vi "Byte_to_DeviceConfigType.vi"(4 "Byte Array":u8[](array[numeric])) -> (1 "output cluster":T1)   [LabVIEW 2016]
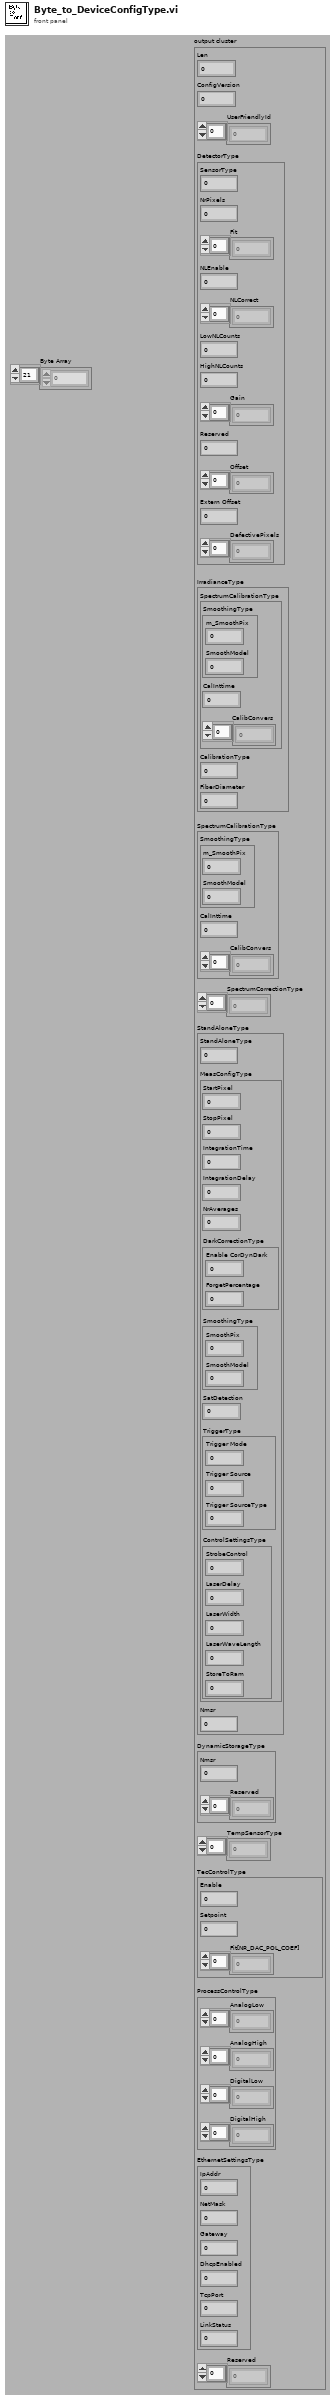
[diagram p1: front panel]
types:
  T1 = cluster{"Len":u16, "ConfigVersion":u16, "UserFriendlyId":u8[], "DetectorType":cluster{"SensorType":u8, "NrPixels":u16, "Fit":sgl[], "NLEnable":u8, "NLCorrect":dbl[], "LowNLCounts":dbl, "HighNLCounts":dbl, "Gain":sgl[], "Reserved":sgl, "Offset":sgl[], "Extern Offset":sgl, "DefectivePixels":u16[]}, "IrradianceType":cluster{"SpectrumCalibrationType":cluster{"SmoothingType":cluster{"m_SmoothPix":u16, "SmoothModel":u8}, "CalInttime":sgl, "CalibConvers":sgl[]}, "CalibrationType":u8, "FiberDiameter":i32}, "SpectrumCalibrationType":cluster{"SmoothingType":cluster{"m_SmoothPix":u16, "SmoothModel":u8}, "CalInttime":sgl, "CalibConvers":sgl[]}, "SpectrumCorrectionType":sgl[], "StandAloneType":cluster{"StandAloneType":u8, "MeasConfigType":cluster{"StartPixel":u16, "StopPixel":u16, "IntegrationTime":sgl, "IntegrationDelay":u32, "NrAverages":u32, "DarkCorrectionType":cluster{"Enable CorDynDark":u8, "ForgetPercentage":u8}, "SmoothingType":cluster{"SmoothPix":u16, "SmoothModel":u8}, "SatDetection":u8, "TriggerType":cluster{"Trigger Mode":u8, "Trigger Source":u8, "Trigger SourceType":u8}, "ControlSettingsType":cluster{"StrobeControl":u16, "LaserDelay":u32, "LaserWidth":u32, "LaserWaveLength":sgl, "StoreToRam":u16}}, "Nmsr":i16}, "DynamicStorageType":cluster{"Nmsr":i32, "Reserved":u8[]}, "TempSensorType":sgl[], "TecControlType":cluster{"Enable":u8, "Setpoint":sgl, "Fit[NR_DAC_POL_COEF]":sgl[]}, "ProcessControlType":cluster{"AnalogLow":sgl[], "AnalogHigh":sgl[], "DigitalLow":sgl[], "DigitalHigh":sgl[]}, "EthernetSettingsType":cluster{"IpAddr":u32, "NetMask":u32, "Gateway":u32, "DhcpEnabled":u8, "TcpPort":u16, "LinkStatus":u8}, "Reserved":u8[]}
  T2 = cluster{"Len":u16, "ConfigVersion":u16, "UserFriendlyId":u8[], "DetectorType":cluster{"SensorType":u8, "NrPixels":u16, "Fit":sgl[], "NLEnable":u8, "NLCorrect":dbl[], "LowNLCounts":dbl, "HighNLCounts":dbl, "Gain":sgl[], "Reserved":sgl, "Offset":sgl[], "Extern Offset":sgl, "DefectivePixels":u16[]}, "IrradianceType":cluster{"SpectrumCalibrationType":cluster{"SmoothingType":cluster{"m_SmoothPix":u16, "SmoothModel":u8}, "CalInttime":sgl, "CalibConvers":sgl[]}, "CalibrationType":u8, "FiberDiameter":i32}, "SpectrumCalibrationType":cluster{"SmoothingType":cluster{"m_SmoothPix":u16, "SmoothModel":u8}, "CalInttime":sgl, "CalibConvers":sgl[]}, "SpectrumCorrectionType":sgl[], "StandAloneType":cluster{"StandAloneType":u8, "MeasConfigType":cluster{"StartPixel":u16, "StopPixel":u16, "IntegrationTime":sgl, "IntegrationDelay":u32, "NrAverages":u32, "DarkCorrectionType":cluster{"Enable CorDynDark":u8, "ForgetPercentage":u8}, "SmoothingType":cluster{"SmoothPix":u16, "SmoothModel":u8}, "SatDetection":u8, "TriggerType":cluster{"Trigger Mode":u8, "Trigger Source":u8, "Trigger SourceType":u8}, "ControlSettingsType":cluster{"StrobeControl":u16, "LaserDelay":u32, "LaserWidth":u32, "LaserWaveLength":sgl, "StoreToRam":u16}}, "Nmsr":i16}, "DynamicStorageType":cluster{"Nmsr":i32, "Reserved":u8[]}, "TempSensorType":sgl[], "TecControlType":cluster{"Enable":u8, "Setpoint":sgl, "Fit[NR_DAC_POL_COEF]":sgl[]}, "ProcessControlType\n":cluster{"AnalogLow":sgl[], "AnalogHigh":sgl[], "DigitalLow":sgl[], "DigitalHigh":sgl[]}, "EthernetSettingsType":cluster{"IpAddr":u32, "NetMask":u32, "Gateway":u32, "DhcpEnabled":u8, "TcpPort":u16, "LinkStatus":u8}, "Reserved":u8[]}
  T3 = cluster{u8, u16, sgl[], u8, dbl[], dbl, dbl, sgl[], sgl, sgl[], sgl, u16[]}
  T4 = cluster{cluster{cluster{u16, u8}, sgl, sgl[]}, u8, i32}
  T5 = cluster{u16, u16, sgl, u32, u32, cluster{u8, u8}, cluster{u16, u8}, u8, cluster{u8, u8, u8}, cluster{u16, u32, u32, sgl, u16}}
  T6 = cluster{u8, cluster{u16, u16, sgl, u32, u32, cluster{u8, u8}, cluster{u16, u8}, u8, cluster{u8, u8, u8}, cluster{u16, u32, u32, sgl, u16}}, i16}
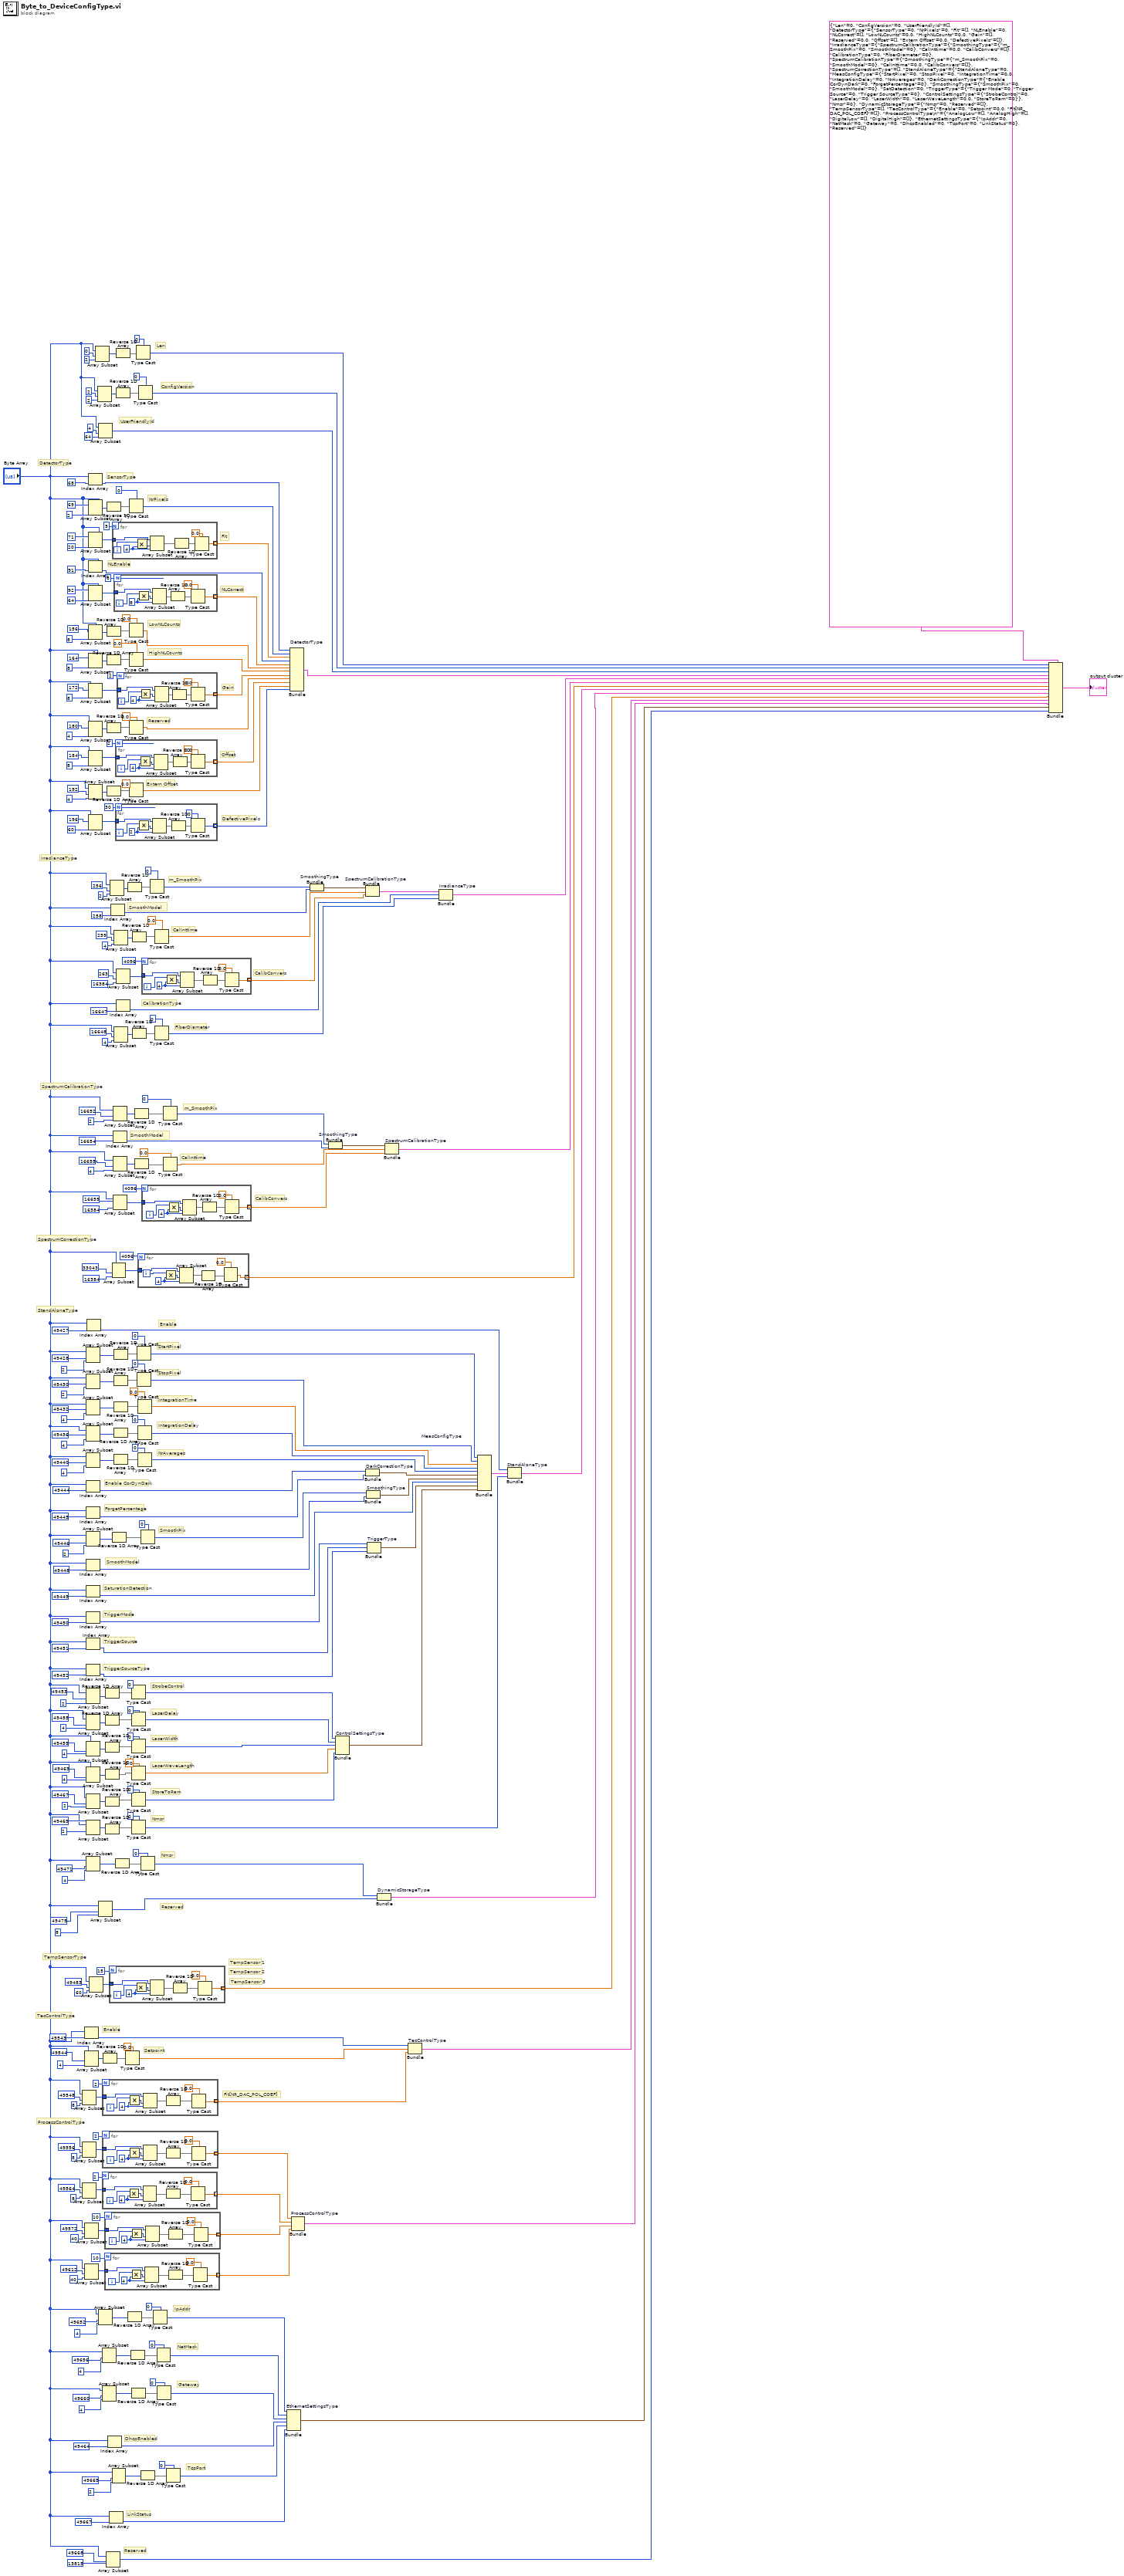
[diagram p0: block diagram]
diagram:
  # "Enable"
  # "LinkStatus"
  # "DhcpEnabled"
  # "TcpPort"
  # "Gateway"
  # "NetMask"
  # "IpAddr"
  # "ProcessControlType"
  # "TecControlType"
  # "Len"
  # "ConfigVersion"
  # "Fit[NR_DAC_POL_COEF]"
  # "Setpoint"
  # "Enable"
  # "UserFriendlyId"
  # "SensorType"
  # "NrPixels"
  # "Fit"
  # "NLEnable"
  # "NLCorrect"
  # "LowNLCounts"
  # "HighNLCounts"
  # "Gain"
  # "Offset"
  # "DetectorType"
  # "TempSensor 3"
  # "TempSensor 2"
  # "Reserved"
  # "TempSensor 1"
  # "TempSensorType"
  # "Reserved"
  # "Nmsr"
  # "Nmsr"
  # "StoreToRam"
  # "LaserWaveLength"
  # "LaserWidth"
  # "LaserDelay"
  # "StrobeControl"
  # "TriggerSourceType"
  # "TriggerSource"
  # "TriggerMode"
  # "SaturationDetection"
  # "SmoothModel"
  # "SmoothPix"
  # "ForgetPercentage"
  # "Enable CorDynDark"
  # "NrAverages"
  # "IntegrationDelay"
  # "IntegrationTime"
  # "StopPixel"
  # "StartPixel"
  # "StandAloneType"
  # "SpectrumCorrectionType"
  # "CalibConvers"
  # "CalInttime"
  # "SmoothModel"
  # "m_SmoothPix"
  # "SpectrumCalibrationType"
  # "FiberDiameter"
  # "CalibrationType"
  # "CalibConvers"
  # "CalInttime"
  # "SmoothModel"
  # "IrradianceType"
  # "m_SmoothPix"
  # "DefectivePixels"
  # "Reserved"
  # "Extern Offset"
  n1 = Array Subset(array="Byte Array", index=49564, length=8) -> (w59:u8[])
  n2 = Array Subset(array="Byte Array", index=49548, length=8) -> (w68:u8[])
  n3 = Array Subset(array="Byte Array", index=49556, length=8) -> (w63:u8[])
  n4 = Index Array(array="Byte Array", index=49543 ("length")) -> (element=w75:u8)
  n5 = Array Subset(array="Byte Array", index=49612, length=40) -> (w51:u8[])
  n6 = Array Subset(array="Byte Array", index=49544, length=4) -> (w71:u8[])
  n7 = Array Subset(array="Byte Array", index=49572, length=40) -> (w55:u8[])
  n8 = Array Subset(array="Byte Array", index=49471 ("length"), length=4) -> (w42:u8[])
  n9 = Array Subset(array="Byte Array", index=49428, length=2) -> (w219:u8[])
  n10 = Array Subset(array="Byte Array", index=49430, length=2) -> (w214:u8[])
  n11 = Array Subset(array="Byte Array", index=49432, length=4) -> (w211:u8[])
  n12 = Array Subset(array="Byte Array", index=49436, length=4) -> (w202:u8[])
  n13 = Array Subset(array="Byte Array", index=49440, length=4) -> (w199:u8[])
  n14 = Index Array(array="Byte Array", index=49444 ("length")) -> (element=w94:u8)
  n15 = Index Array(array="Byte Array", index=49445 ("length")) -> (element=w93:u8)
  n16 = Array Subset(array="Byte Array", index=49446, length=2) -> (w193:u8[])
  n17 = Index Array(array="Byte Array", index=49448 ("length")) -> (element=w91:u8)
  n18 = Index Array(array="Byte Array", index=49449 ("length")) -> (element=w90:u8)
  n19 = Index Array(array="Byte Array", index=49450 ("length")) -> (element=w89:u8)
  n20 = Index Array(array="Byte Array", index=49451 ("length")) -> (element=w88:u8)
  n21 = Index Array(array="Byte Array", index=49452 ("length")) -> (element=w87:u8)
  n22 = Array Subset(array="Byte Array", index=49453, length=2) -> (w181:u8[])
  n23 = Array Subset(array="Byte Array", index=49455, length=4) -> (w178:u8[])
  n24 = Array Subset(array="Byte Array", index=49459, length=4) -> (w171:u8[])
  n25 = Array Subset(array="Byte Array", index=49463, length=4) -> (w168:u8[])
  n26 = Array Subset(array="Byte Array", index=49467, length=2) -> (w161:u8[])
  n27 = Array Subset(array="Byte Array", index=49469, length=2) -> (w156:u8[])
  n28 = Index Array(array="Byte Array", index=49427 ("length")) -> (element=w100:u8)
  n29 = Index Array(array="Byte Array", index=68 ("length")) -> (element=w133:u8)
  n30 = Array Subset(array="Byte Array", index=69, length=2) -> (w297:u8[])
  n31 = Array Subset(array="Byte Array", index=71, length=20) -> (w130:u8[])
  n32 = Index Array(array="Byte Array", index=91 ("length")) -> (element=w129:u8)
  n33 = Array Subset(array="Byte Array", index=92, length=64) -> (w127:u8[])
  n34 = Array Subset(array="Byte Array", index=156, length=8) -> (w283:u8[])
  n35 = Array Subset(array="Byte Array", index=164, length=8) -> (w280:u8[])
  n36 = Array Subset(array="Byte Array", index=172, length=8) -> (w123:u8[])
  n37 = Array Subset(array="Byte Array", index=180, length=4) -> (w271:u8[])
  n38 = Array Subset(array="Byte Array", index=184, length=8) -> (w120:u8[])
  n39 = Array Subset(array="Byte Array", index=192, length=4) -> (w263:u8[])
  n40 = Array Subset(array="Byte Array", index=196, length=60) -> (w118:u8[])
  n41 = Array Subset(array="Byte Array", index=49483, length=60) -> (w78:u8[])
  n42 = Array Subset(array="Byte Array", index=0, length=2) -> (w302:u8[])
  n43 = Array Subset(array="Byte Array", index=2, length=2) -> (w301:u8[])
  n44 = Array Subset(array="Byte Array", index=4, length=64) -> (w134:u8[])
  n45 = Array Subset(array="Byte Array", index=49475, length=8) -> (w77:u8[])
  n46 = Array Subset(array="Byte Array", index=49652 ("length"), length=4) -> (w35:u8[])
  n47 = for {
    N: 2 -> [_]
    tunnel: w59 -> [w315]
    tunnel: [w313] -> w46 mode=indexing
    i -> [w316]
    w317 = 4 ("length")
    n48 = Multiply(x=w316, y=w317) -> (x*y=w318:i32)
    n49 = Array Subset(array=w315, index=w318, length=w317) -> (w311:u8[])
    n50 = Reverse 1D Array(array=w311) -> (reversed array=w312:u8[])
    n51 = Type Cast(type=sgl 0.0, x=w312) -> (*(type *) &x=w313:sgl)
  }
  n52 = Array Subset(array="Byte Array", index=49656 ("length"), length=4) -> (w30:u8[])
  n53 = for {
    N: 2 -> [_]
    tunnel: w68 -> [w323]
    tunnel: [w321] -> w64 mode=indexing
    i -> [w324]
    w325 = 4 ("length")
    n54 = Multiply(x=w324, y=w325) -> (x*y=w326:i32)
    n55 = Array Subset(array=w323, index=w326, length=w325) -> (w319:u8[])
    n56 = Reverse 1D Array(array=w319) -> (reversed array=w320:u8[])
    n57 = Type Cast(type=sgl 0.0, x=w320) -> (*(type *) &x=w321:sgl)
  }
  n58 = for {
    N: 2 -> [_]
    tunnel: w63 -> [w331]
    tunnel: [w329] -> w47 mode=indexing
    i -> [w332]
    w333 = 4 ("length")
    n59 = Multiply(x=w332, y=w333) -> (x*y=w334:i32)
    n60 = Array Subset(array=w331, index=w334, length=w333) -> (w327:u8[])
    n61 = Reverse 1D Array(array=w327) -> (reversed array=w328:u8[])
    n62 = Type Cast(type=sgl 0.0, x=w328) -> (*(type *) &x=w329:sgl)
  }
  n63 = Array Subset(array="Byte Array", index=49660 ("length"), length=4) -> (w25:u8[])
  n64 = Reverse 1D Array(array=w71) -> (reversed array=w70:u8[])
  n65 = for {
    N: 10 -> [_]
    tunnel: w51 -> [w339]
    tunnel: [w337] -> w44 mode=indexing
    i -> [w340]
    w341 = 4 ("length")
    n66 = Multiply(x=w340, y=w341) -> (x*y=w342:i32)
    n67 = Array Subset(array=w339, index=w342, length=w341) -> (w335:u8[])
    n68 = Reverse 1D Array(array=w335) -> (reversed array=w336:u8[])
    n69 = Type Cast(type=sgl 0.0, x=w336) -> (*(type *) &x=w337:sgl)
  }
  n70 = for {
    N: 10 -> [_]
    tunnel: w55 -> [w347]
    tunnel: [w345] -> w45 mode=indexing
    i -> [w348]
    w349 = 4 ("length")
    n71 = Multiply(x=w348, y=w349) -> (x*y=w350:i32)
    n72 = Array Subset(array=w347, index=w350, length=w349) -> (w343:u8[])
    n73 = Reverse 1D Array(array=w343) -> (reversed array=w344:u8[])
    n74 = Type Cast(type=sgl 0.0, x=w344) -> (*(type *) &x=w345:sgl)
  }
  n75 = Reverse 1D Array(array=w181) -> (reversed array=w180:u8[])
  n76 = Reverse 1D Array(array=w178) -> (reversed array=w179:u8[])
  n77 = Reverse 1D Array(array=w171) -> (reversed array=w170:u8[])
  n78 = Reverse 1D Array(array=w168) -> (reversed array=w169:u8[])
  n79 = Reverse 1D Array(array=w161) -> (reversed array=w162:u8[])
  n80 = Reverse 1D Array(array=w156) -> (reversed array=w155:u8[])
  n81 = Array Subset(array="Byte Array", index=49668, length=13815) -> (w7:u8[])
  n82 = Reverse 1D Array(array=w297) -> (reversed array=w298:u8[])
  n83 = Reverse 1D Array(array=w283) -> (reversed array=w282:u8[])
  n84 = Reverse 1D Array(array=w280) -> (reversed array=w281:u8[])
  n85 = Reverse 1D Array(array=w271) -> (reversed array=w270:u8[])
  n86 = Reverse 1D Array(array=w263) -> (reversed array=w264:u8[])
  n87 = Index Array(array="Byte Array", index=49464 ("length")) -> (element=w10:u8)
  n88 = for {
    N: 15 -> [_]
    tunnel: w78 -> [w355]
    tunnel: [w353] -> w3 mode=indexing
    i -> [w356]
    w357 = 4 ("length")
    n89 = Multiply(x=w356, y=w357) -> (x*y=w358:i32)
    n90 = Array Subset(array=w355, index=w358, length=w357) -> (w351:u8[])
    n91 = Reverse 1D Array(array=w351) -> (reversed array=w352:u8[])
    n92 = Type Cast(type=sgl 0.0, x=w352) -> (*(type *) &x=w353:sgl)
  }
  n93 = Index Array(array="Byte Array", index=49667 ("length")) -> (element=w8:u8)
  n94 = Array Subset(array="Byte Array", index=256, length=2) -> (w254:u8[])
  n95 = Index Array(array="Byte Array", index=258 ("length")) -> (element=w115:u8)
  n96 = for {
    N: 5 -> [_]
    tunnel: w130 -> [w363]
    tunnel: [w361] -> w131 mode=indexing
    i -> [w364]
    w365 = 4 ("length")
    n97 = Multiply(x=w364, y=w365) -> (x*y=w366:i32)
    n98 = Array Subset(array=w363, index=w366, length=w365) -> (w360:u8[])
    n99 = Reverse 1D Array(array=w360) -> (reversed array=w359:u8[])
    n100 = Type Cast(type=sgl 0.0, x=w359) -> (*(type *) &x=w361:sgl)
  }
  n101 = Array Subset(array="Byte Array", index=33043, length=16384) -> (w86:u8[])
  n102 = Array Subset "Array Subset"(array="Byte Array", index=49665 ("length"), length=2) -> (w17:u8[])
  n103 = Reverse 1D Array(array=w193) -> (reversed array=w194:u8[])
  n104 = Array Subset(array="Byte Array", index=16652, length=2) -> (w228:u8[])
  n105 = Index Array(array="Byte Array", index=16654 ("length")) -> (element=w107:u8)
  n106 = Array Subset(array="Byte Array", index=16655, length=4) -> (w231:u8[])
  n107 = Array Subset(array="Byte Array", index=16659, length=16384) -> (w85:u8[])
  n108 = Reverse 1D Array(array=w219) -> (reversed array=w220:u8[])
  n109 = Reverse 1D Array(array=w214) -> (reversed array=w213:u8[])
  n110 = Reverse 1D Array(array=w211) -> (reversed array=w212:u8[])
  n111 = Reverse 1D Array(array=w202) -> (reversed array=w201:u8[])
  n112 = Reverse 1D Array(array=w199) -> (reversed array=w200:u8[])
  n113 = for {
    N: 8 -> [_]
    tunnel: w127 -> [w371]
    tunnel: [w369] -> w128 mode=indexing
    i -> [w372]
    w373 = 8 ("length")
    n114 = Multiply(x=w372, y=w373) -> (x*y=w374:i32)
    n115 = Array Subset(array=w371, index=w374, length=w373) -> (w368:u8[])
    n116 = Reverse 1D Array(array=w368) -> (reversed array=w367:u8[])
    n117 = Type Cast(type=0.0, x=w367) -> (*(type *) &x=w369:dbl)
  }
  n118 = Array Subset(array="Byte Array", index=259, length=4) -> (w250:u8[])
  n119 = Array Subset(array="Byte Array", index=16648, length=4) -> (w241:u8[])
  n120 = for {
    N: 30 -> [_]
    tunnel: w118 -> [w379]
    tunnel: [w377] -> w117 mode=indexing
    i -> [w380]
    w381 = 2 ("length")
    n121 = Multiply(x=w380, y=w381) -> (x*y=w382:i32)
    n122 = Array Subset(array=w379, index=w382, length=w381) -> (w376:u8[])
    n123 = Reverse 1D Array(array=w376) -> (reversed array=w375:u8[])
    n124 = Type Cast(type=u16 0, x=w375) -> (*(type *) &x=w377:u16)
  }
  n125 = Reverse 1D Array(array=w42) -> (reversed array=w43:u8[])
  n126 = for {
    N: 2 -> [_]
    tunnel: w120 -> [w387]
    tunnel: [w385] -> w121 mode=indexing
    i -> [w388]
    w389 = 4 ("length")
    n127 = Multiply(x=w388, y=w389) -> (x*y=w390:i32)
    n128 = Array Subset(array=w387, index=w390, length=w389) -> (w384:u8[])
    n129 = Reverse 1D Array(array=w384) -> (reversed array=w383:u8[])
    n130 = Type Cast(type=sgl 0.0, x=w383) -> (*(type *) &x=w385:sgl)
  }
  n131 = Array Subset(array="Byte Array", index=263, length=16384) -> (w113:u8[])
  n132 = Reverse 1D Array(array=w302) -> (reversed array=w145:u8[])
  n133 = Reverse 1D Array(array=w301) -> (reversed array=w300:u8[])
  n134 = Index Array(array="Byte Array", index=16647 ("length")) -> (element=w111:u8)
  n135 = for {
    N: 2 -> [_]
    tunnel: w123 -> [w395]
    tunnel: [w393] -> w124 mode=indexing
    i -> [w396]
    w397 = 4 ("length")
    n136 = Multiply(x=w396, y=w397) -> (x*y=w398:i32)
    n137 = Array Subset(array=w395, index=w398, length=w397) -> (w392:u8[])
    n138 = Reverse 1D Array(array=w392) -> (reversed array=w391:u8[])
    n139 = Type Cast(type=sgl 0.0, x=w391) -> (*(type *) &x=w393:sgl)
  }
  n140 = Type Cast(type=sgl 0.0, x=w70) -> (*(type *) &x=w69:sgl)
  n141 = Reverse 1D Array(array=w35) -> (reversed array=w36:u8[])
  n142 = Reverse 1D Array(array=w254) -> (reversed array=w253:u8[])
  n143 = Type Cast(type=u16 0, x=w298) -> (*(type *) &x=w132:u16)
  n144 = Type Cast(type=0.0, x=w282) -> (*(type *) &x=w126:dbl)
  n145 = Type Cast(type=0.0, x=w281) -> (*(type *) &x=w125:dbl)
  n146 = Type Cast(type=sgl 0.0, x=w270) -> (*(type *) &x=w122:sgl)
  n147 = Type Cast(type=sgl 0.0, x=w264) -> (*(type *) &x=w119:sgl)
  n148 = Reverse 1D Array(array=w30) -> (reversed array=w31:u8[])
  n149 = Type Cast(type=u16 0, x=w180) -> (*(type *) &x=w84:u16)
  n150 = Type Cast(type=u32 0, x=w179) -> (*(type *) &x=w83:u32)
  n151 = Type Cast(type=u32 0, x=w170) -> (*(type *) &x=w82:u32)
  n152 = Type Cast(type=sgl 0.0, x=w169) -> (*(type *) &x=w81:sgl)
  n153 = Type Cast(type=u16 0, x=w162) -> (*(type *) &x=w80:u16)
  n154 = Type Cast(type=i16 0, x=w155) -> (*(type *) &x=w79:i16)
  n155 = Reverse 1D Array(array=w25) -> (reversed array=w26:u8[])
  n156 = Reverse 1D Array(array=w250) -> (reversed array=w251:u8[])
  n157 = Reverse 1D Array(array=w241) -> (reversed array=w242:u8[])
  n158 = Reverse 1D Array(array=w228) -> (reversed array=w146:u8[])
  n159 = Reverse 1D Array(array=w231) -> (reversed array=w230:u8[])
  n160 = Type Cast(type=u16 0, x=w145) -> (*(type *) &x=w136:u16)
  n161 = Type Cast(type=u16 0, x=w220) -> (*(type *) &x=w99:u16)
  n162 = Type Cast(type=u16 0, x=w213) -> (*(type *) &x=w98:u16)
  n163 = Type Cast(type=sgl 0.0, x=w212) -> (*(type *) &x=w97:sgl)
  n164 = Type Cast(type=u32 0, x=w201) -> (*(type *) &x=w96:u32)
  n165 = Type Cast(type=u32 0, x=w200) -> (*(type *) &x=w95:u32)
  n166 = for {
    N: 4096 -> [_]
    tunnel: w86 -> [w403]
    tunnel: [w401] -> w102 mode=indexing
    i -> [w404]
    w405 = 4 ("length")
    n167 = Multiply(x=w404, y=w405) -> (x*y=w406:i32)
    n168 = Array Subset(array=w403, index=w406, length=w405) -> (w400:u8[])
    n169 = Reverse 1D Array(array=w400) -> (reversed array=w399:u8[])
    n170 = Type Cast(type=sgl 0.0, x=w399) -> (*(type *) &x=w401:sgl)
  }
  n171 = Type Cast(type=u16 0, x=w300) -> (*(type *) &x=w135:u16)
  n172 = Type Cast(type=u32 0, x=w43) -> (*(type *) &x=w39:u32)
  n173 = Type Cast(type=u16 0, x=w194) -> (*(type *) &x=w92:u16)
  n174 = Reverse 1D Array(array=w17) -> (reversed array=w18:u8[])
  n175 = for {
    N: 4096 -> [_]
    tunnel: w113 -> [w411]
    tunnel: [w409] -> w112 mode=indexing
    i -> [w412]
    w413 = 4 ("length")
    n176 = Multiply(x=w412, y=w413) -> (x*y=w414:i32)
    n177 = Array Subset(array=w411, index=w414, length=w413) -> (w408:u8[])
    n178 = Reverse 1D Array(array=w408) -> (reversed array=w407:u8[])
    n179 = Type Cast(type=sgl 0.0, x=w407) -> (*(type *) &x=w409:sgl)
  }
  n180 = for {
    N: 4096 -> [_]
    tunnel: w85 -> [w419]
    tunnel: [w417] -> w105 mode=indexing
    i -> [w420]
    w421 = 4 ("length")
    n181 = Multiply(x=w420, y=w421) -> (x*y=w422:i32)
    n182 = Array Subset(array=w419, index=w422, length=w421) -> (w416:u8[])
    n183 = Reverse 1D Array(array=w416) -> (reversed array=w415:u8[])
    n184 = Type Cast(type=sgl 0.0, x=w415) -> (*(type *) &x=w417:sgl)
  }
  n185 = Type Cast(type=u16 0, x=w253) -> (*(type *) &x=w116:u16)
  n186 = Type Cast(type=u32 0, x=w36) -> (*(type *) &x=w21:u32)
  n187 = Type Cast(type=sgl 0.0, x=w251) -> (*(type *) &x=w114:sgl)
  n188 = Type Cast(type=0, x=w242) -> (*(type *) &x=w110:i32)
  n189 = Type Cast(type=u32 0, x=w31) -> (*(type *) &x=w20:u32)
  n190 = Type Cast(type=u32 0, x=w26) -> (*(type *) &x=w19:u32)
  n191 = Type Cast(type=u16 0, x=w146) -> (*(type *) &x=w108:u16)
  n192 = Type Cast(type=sgl 0.0, x=w230) -> (*(type *) &x=w106:sgl)
  n193 = Type Cast(type=u16 0, x=w18) -> (*(type *) &x=w9:u16)
  n194 = Bundle "EthernetSettingsType"(w21, w20, w19, w10, w9, w8) -> (w6:cluster{u32, u32, u32, u8, u16, u8})  [unwired: 1 in]
  n195 = Bundle "DetectorType"(w133, w132, w131, w129, w128, w126, w125, w124, w122, w121, w119, w117) -> (w144:T3)  [unwired: 1 in]
  n196 = Bundle "ProcessControlType"(w47, w46, w45, w44) -> (w5:cluster{sgl[], sgl[], sgl[], sgl[]})  [unwired: 1 in]
  n197 = Bundle "SmoothingType"(w116, w115) -> (w139:cluster{u16, u8})  [unwired: 1 in]
  n198 = Bundle "SmoothingType"(w108, w107) -> (w109:cluster{u16, u8})  [unwired: 1 in]
  n199 = Bundle "ControlSettingsType"(w84, w83, w82, w81, w80) -> (w137:cluster{u16, u32, u32, sgl, u16})  [unwired: 1 in]
  n200 = Bundle "SpectrumCalibrationType"(w139, w114, w112) -> (w104:cluster{cluster{u16, u8}, sgl, sgl[]})  [unwired: 1 in]
  n201 = Bundle "DarkCorrectionType"(w94, w93) -> (w140:cluster{u8, u8})  [unwired: 1 in]
  n202 = Bundle "SmoothingType"(w92, w91) -> (w101:cluster{u16, u8})  [unwired: 1 in]
  n203 = Bundle "TriggerType"(w89, w88, w87) -> (w138:cluster{u8, u8, u8})  [unwired: 1 in]
  n204 = Bundle "DynamicStorageType"(w39, w77) -> (w2:cluster{u32, u8[]})  [unwired: 1 in]
  n205 = Bundle "SpectrumCalibrationType"(w109, w106, w105) -> (w103:cluster{cluster{u16, u8}, sgl, sgl[]})  [unwired: 1 in]
  n206 = Bundle "TecControlType"(w75, w69, w64) -> (w4:cluster{u8, sgl, sgl[]})  [unwired: 1 in]
  n207 = Bundle "IrradianceType"(w104, w111, w110) -> (w143:T4)  [unwired: 1 in]
  n208 = Bundle "MeasConfigType"(w99, w98, w97, w96, w95, w140, w101, w90, w138, w137) -> (w141:T5)  [unwired: 1 in]
  n209 = Bundle "StandAloneType"(w100, w141, w79) -> (w142:T6)  [unwired: 1 in]
  n210 = Bundle(cluster=T2 {"Len"=0, "ConfigVersion"=0, "UserFriendlyId"=[], "DetectorType"={"SensorType"=0, "NrPixels"=0, "Fit"=[], "NLEnable"=0, "NLCorrect"=[], "LowNLCounts"=0.0, "HighNLCounts"=0.0, "Gain"=[], "Reserved"=0.0, "Offset"=[], "Extern Offset"=0.0, "DefectivePixels"=[]}, "IrradianceType"={"SpectrumCalibrationType"={"SmoothingType"={"m_SmoothPix"=0, "SmoothModel"=0}, "CalInttime"=0.0, "CalibConvers"=[]}, "CalibrationType"=0, "FiberDiameter"=0}, "SpectrumCalibrationType"={"SmoothingType"={"m_SmoothPix"=0, "SmoothModel"=0}, "CalInttime"=0.0, "CalibConvers"=[]}, "SpectrumCorrectionType"=[], "StandAloneType"={"StandAloneType"=0, "MeasConfigType"={"StartPixel"=0, "StopPixel"=0, "IntegrationTime"=0.0, "IntegrationDelay"=0, "NrAverages"=0, "DarkCorrectionType"={"Enable CorDynDark"=0, "ForgetPercentage"=0}, "SmoothingType"={"SmoothPix"=0, "SmoothModel"=0}, "SatDetection"=0, "TriggerType"={"Trigger Mode"=0, "Trigger Source"=0, "Trigger SourceType"=0}, "ControlSettingsType"={"StrobeControl"=0, "LaserDelay"=0, "LaserWidth"=0, "LaserWaveLength"=0.0, "StoreToRam"=0}}, "Nmsr"=0}, "DynamicStorageType"={"Nmsr"=0, "Reserved"=[]}, "TempSensorType"=[], "TecControlType"={"Enable"=0, "Setpoint"=0.0, "Fit[NR_DAC_POL_COEF]"=[]}, "ProcessControlType\n"={"AnalogLow"=[], "AnalogHigh"=[], "DigitalLow"=[], "DigitalHigh"=[]}, "EthernetSettingsType"={"IpAddr"=0, "NetMask"=0, "Gateway"=0, "DhcpEnabled"=0, "TcpPort"=0, "LinkStatus"=0}, "Reserved"=[]} ("DeviceConfig"), "Len"=w136, "ConfigVersion"=w135, "UserFriendlyId"=w134, "DetectorType"=w144, "IrradianceType"=w143, "SpectrumCalibrationType"=w103, "SpectrumCorrectionType"=w102, "StandAloneType"=w142, "DynamicStorageType"=w2, "TempSensorType"=w3, "TecControlType"=w4, "ProcessControlType"=w5, "EthernetSettingsType"=w6, "Reserved"=w7) -> (→"output cluster":T2)
